vi "Torque, Load, and Efficiency (Air Gap, N Motors).vi"(0 "phase voltage waveforms":waveform(dbl)[](array[waveform]), 1 "fundamental frequency [Hz]":dbl=50.0, 2 "reset? (F)":bool, 5 "current waveforms":waveform(dbl)[](array[waveform]), 7 "speed [RPM]":dbl[](array[numeric]), 11 "error in (no error)":errorcluster, 12 "nameplate information":T1, 13 "total input active power [W]":dbl[](array[numeric]), 14 "stator resistance [ohms]":dbl[](array[numeric])) -> (3 "torque waveforms [Nm]":waveform(dbl)[](array[waveform]), 4 "torque [Nm]":dbl[](array[numeric]), 6 "load [kW]":dbl[](array[numeric]), 8 "efficiency [%]":dbl[](array[numeric]), 15 "error out":errorcluster)   [LabVIEW 2014, in "NI_EP_Motor Monitoring.lvlib"]
doc: "Calculates the torque, load, and efficiency values based on the motor nameplate information. You must manually select the polymorphic instance you want to use."
uses:
  <vilib>/addons/Electrical Power/Motor Monitoring/NI_EP_Motor Monitoring.lvlib
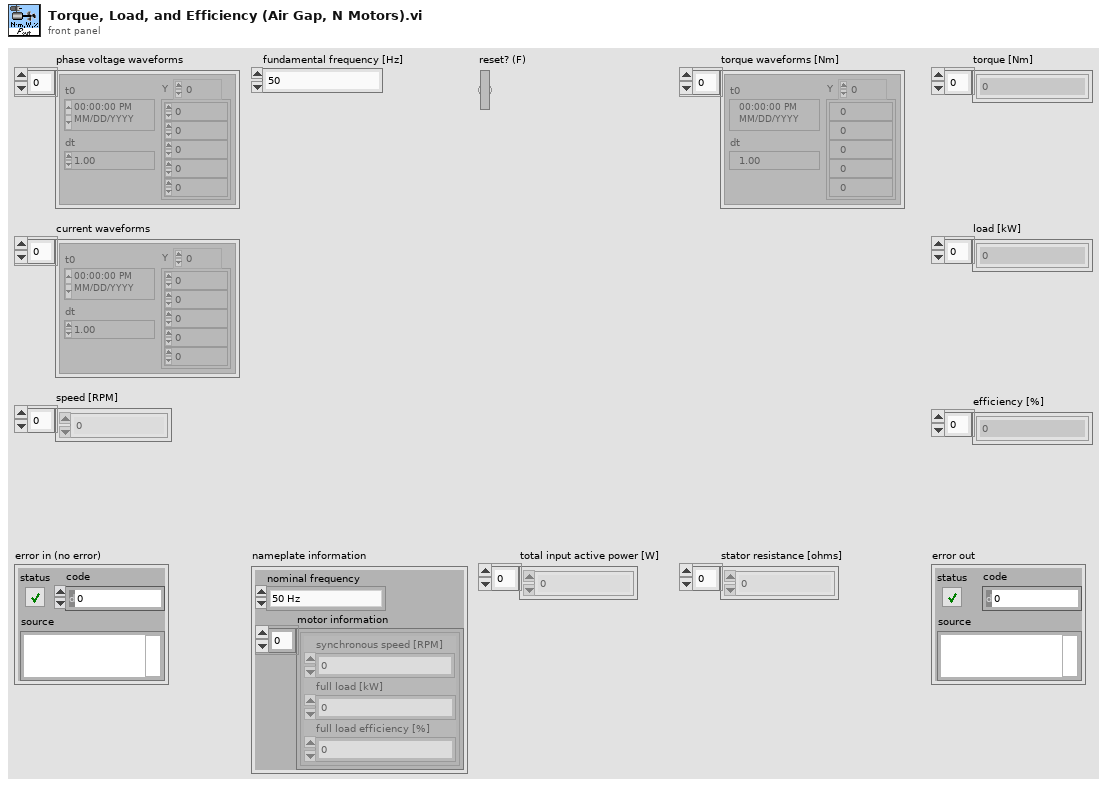
[diagram p1: front panel]
types:
  T1 = cluster{"nominal frequency":enum16{"50 Hz", "60 Hz"}, "motor information":cluster{"synchronous speed [RPM]":dbl, "full load [kW]":dbl, "full load efficiency [%]":dbl}[]}
  T2 = cluster{"synchronous speed [RPM]":dbl, "full load [kW]":dbl, "full load efficiency [%]":dbl}[]
  T3 = typedef "NI_EP_Motor Monitoring.lvlib/ep_Initial Conditions for Air Gap.ctl" = cluster{"integration state in A":cluster{"initial value":dbl, "initial integration":dbl}, "integration state in B":cluster{"initial value":dbl, "initial integration":dbl}, "integrated state A":dbl[], "integrated state B":dbl[], "previous length":i32, "loss and polepair":cluster{"Pstray [W]":dbl, "Pfric [W]":dbl, "Polepair #":i32, "synchronous speed [RPM]":dbl}, "expected timestamp":timestamp}
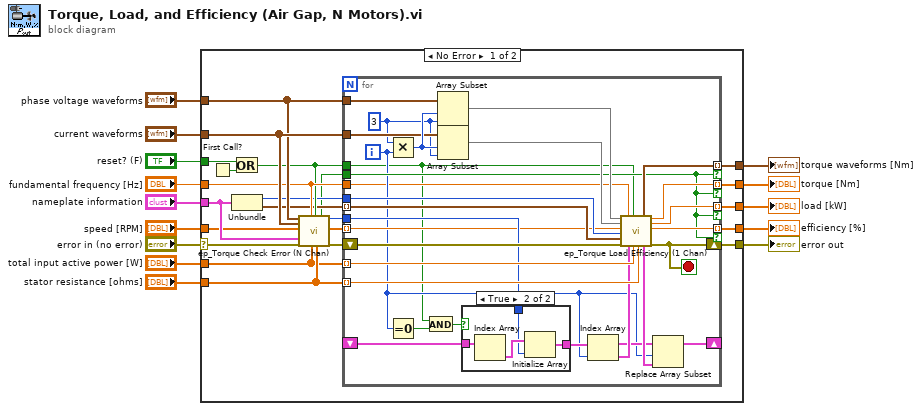
[diagram p0: block diagram]
diagram:
  n1 = case shown="No Error" "error in (no error)" {
    selector: "error in (no error)" -> [w36 w71]
    tunnel: [w21 w71] -> w13
    tunnel: "reset? (F)" -> [w34 _]
    tunnel: "stator resistance [ohms]" -> [w32 _]
    tunnel: "total input active power [W]" -> [w31 _]
    tunnel: "fundamental frequency [Hz]" -> [w26 _]
    tunnel: "nameplate information" -> [w28 _]
    tunnel: "speed [RPM]" -> [w27 _]
    tunnel: "current waveforms" -> [w30 _]
    tunnel: "phase voltage waveforms" -> [w29 _]
    tunnel: [w18 _] -> w4
    tunnel: [w17 _] -> w3
    tunnel: [w16 _] -> w2
    tunnel: [w15 _] -> w1
    frame No Error {
      n2 = First Call?() -> (First Call?: T/F=w35:bool)
      n3 = Or(x=w34, y=w35) -> (x .or. y?=w25:bool)
      n4 = Unbundle(w28) -> ("nominal frequency"=w24:enum16{"50 Hz", "60 Hz"}, "motor information"=w23:T2)
      n5 = call <vilib>:"ep_Torque Check Error (N Chan).vi"("phase voltage waveforms"=w29, "current waveforms"=w30, "speed in [RPM]"=w27, "nameplate information"=w28, "error in (no error)"=w36, "fundamental frequency [Hz]"=w26, "total input active power [W]"=w31, "reset? (F)"=w25, "stator resistance  [ohms]"=w32) -> ("non-empty speed?"=w19:bool, "motor #"=w22:i32, "speed out [RPM]"=w20:dbl[], "error out"=w33:errorcluster)  [unwired: 7 in]
      n6 = for {
        shift-right: [w41] -> w21
        shift-left: w33 -> [w62]
        shift-right: [w48] -> _
        shift-left: _ -> [w46]
        tunnel: w32 -> [w56] mode=indexing
        tunnel: w31 -> [w57] mode=indexing
        tunnel: w30 -> [w64]
        tunnel: w29 -> [w63]
        tunnel: w26 -> [w38]
        tunnel: w25 -> [w37]
        tunnel: w24 -> [w58]
        tunnel: w23 -> [w59] mode=indexing
        tunnel: [w55] -> w15 mode=indexing if=w40
        tunnel: [w54] -> w17 mode=indexing if=w40
        tunnel: [w53] -> w18 mode=indexing if=w40
        tunnel: w22 -> [w45]
        tunnel: w20 -> [w43] mode=indexing
        tunnel: [w42] -> w16 mode=indexing if=w40
        tunnel: w19 -> [w40]
        i -> [w39]
        stop <- w41 stop-if-true
        w52 = 3
        n7 = Multiply(x=w52, y=w39) -> (x*y=w65:i32)
        n8 = Equal To 0?(x=w39) -> (x = 0?=w51:bool)
        n9 = And(x=w37, y=w51) -> (x .and. y?=w47:bool)
        n10 = Array Subset(array=w63, index=w65, length=w52) -> (w61:waveform(dbl)[])
        n11 = Array Subset(array=w64, index=w65, length=w52) -> (w60:waveform(dbl)[])
        n12 = case shown="True" w47 {
          tunnel: w46 -> [w66 w70]
          tunnel: w45 -> [_ w68]
          tunnel: [w66 w67] -> w44
          frame False {
          }
          frame True {
            n13 = Index Array(array=w70) -> (element=w69:T3)  [unwired: 1 in]
            n14 = Initialize Array(w69, w68) -> (w67:T3[])
          }
        }
        n15 = Index Array(array=w44, index=w39) -> (element=w50:T3)
        n16 = call <vilib>:"ep_Torque Load Efficiency (1 Chan).vi"("phase voltage waveforms"=w61, "current waveforms"=w60, "speed [RPM]"=w43, "nominal frequency"=w58, "motor information"=w59, "error in (no error)"=w62, "fundamental frequency [Hz]"=w38, "initial conditions"=w50, "reset? (F)"=w37, "total input active power [W]"=w57, "stator resistance [ohms]"=w56) -> ("torque waveform [Nm]"=w53:waveform(dbl), "final conditions"=w49:T3, "torque [Nm]"=w54:dbl, "load [kW]"=w42:dbl, "efficiency [%]"=w55:dbl, "error out"=w41:errorcluster)  [unwired: 3 in]
        n17 = Replace Array Subset(array=w44, new element=w49, index=w39) -> (w48:T3[])
      }
    }
    frame Error {
    }
  }
  "error out" <- w13
  "torque waveforms [Nm]" <- w4
  "efficiency [%]" <- w1
  "torque [Nm]" <- w3
  "load [kW]" <- w2
